vi "Teleop.vi"(10 "Match Info":T1={"Autonomous Elapsed Seconds"=0.0, "TeleOp Elapsed Seconds"=0.0, "Disabled Elapsed Seconds"=0.0, "Visited Autonomous"=FALSE, "Visited TeleOp"=FALSE, "Visited Disabled"=FALSE, "Autonomous Settings"={"Autonomous Style"=enum."Independent", "VI Refnum"=refnum}}, 11 "Call Context":T2) -> ()   [LabVIEW 2020]
doc: "This VI is called for each TeleOp packet received from the DS where the robot is not disabled. It is often used to read from the joysticks and update I/O or to update setpoints for timed control loops. It should complete and return within 20 milliseconds or it may miss DS packets."
uses:
  <vilib>/Rock Robotics/Network Tables/NT Write Numeric Array.vi
  <vilib>/Rock Robotics/Network Tables/NT Write Boolean Array.vi
  <vilib>/Rock Robotics/WPI/Joystick/XBox Buttons Indexer.ctl
  <vilib>/Rock Robotics/WPI/DriverStation/WPI_DriverStationMatch Info.ctl
  <vilib>/Rock Robotics/WPI/DriverStation/WPI_DriverStationDerivedRobotMode.ctl
panel:
  out "Right  Bumper?":bool
  out "Button  Y?":bool
  out "Button  X?":bool
  out "Button  B?":bool
  out "Left Bumper ?":bool
  out "Button A?":bool
  out "Motor Values":dbl[](array[numeric])
  out "Stick 2":dbl
  out "Stick 1":dbl
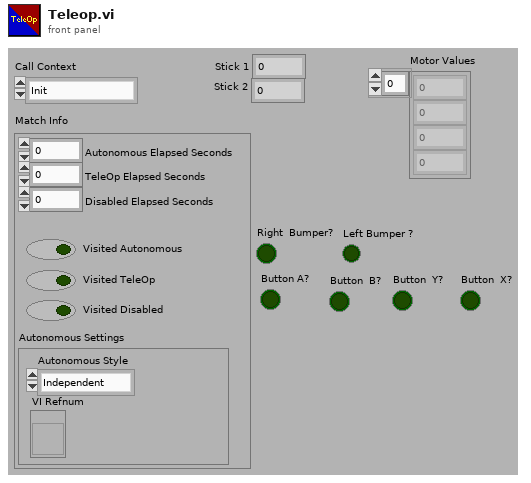
[diagram p1: front panel]
types:
  T1 = typedef "WPI_DriverStationMatch Info.ctl" = cluster{"Autonomous Elapsed Seconds":dbl, "TeleOp Elapsed Seconds":dbl, "Disabled Elapsed Seconds":dbl, "Visited Autonomous":bool, "Visited TeleOp":bool, "Visited Disabled":bool, "Autonomous Settings":cluster{"Autonomous Style":enum16{"Iterative", "Independent"}, "VI Refnum":refnum<vi>}}
  T2 = typedef "WPI_DriverStationDerivedRobotMode.ctl" = enum16{"Init", "Execute", "Stop"}
  T3 = typedef "XBox Buttons Indexer.ctl" = enum16{"A", "B", "X", "Y", "Left Bumper", "Right Bumper", "Back", "Start", "Left Joystick", "Right Joystick"}
  T4 = typedef "WPI_RobotDriveDevRef.ctl" = cluster{"DevStatus":errorcluster, "Motors[]":T5[], "Square Inputs":bool, "Max Output":dbl}
  T5 = typedef "WPI_MotorControlDeviceRef.ctl" = cluster{"DeviceStatus":errorcluster, "Type":T6, "PWM":cluster{"PWM Channel":T7, "DeadBand":T8}, "CAN":cluster{"Device Number":u8, "SetOutput VI Ref":variant, "GetOutput VI Ref":variant, "Enable VI Ref":variant, "Disable VI Ref":variant, "Data":variant}, "Invert":bool, "DIO PWM":cluster{"PWM \"Enable\" Channel":T7, "DIOChannel":T9, "PWM Rate":dbl}}
  T6 = typedef "WPI_MotorControlType.ctl" = enum16{"PWM", "CAN", "DIO PWM"}
  T7 = typedef "FPGA_DIOPWMChannel.ctl" = enum8{"PWM 0", "PWM 1", "PWM 2", "PWM 3", "PWM 4", "PWM 5", "PWM 6", "PWM 7", "PWM 8", "PWM 9", "PWM MXP 0", "PWM MXP 1", "PWM MXP 2", "PWM MXP 3", "PWM MXP 4", "PWM MXP 5", "PWM MXP 6", "PWM MXP 7", "PWM MXP 8", "PWM MXP 9", "Invalid"}
  T8 = typedef "WPI_PWMDeadband.ctl" = cluster{"Name":string, "maxPositivePwm":i32, "minPositivePwm":i32, "centerPwm":i32, "maxNegativePwm":i32, "minNegativePwm":i32, "angularRange":u16}
  T9 = typedef "FPGA_DIOChannel.ctl" = enum8{"DIO 0", "DIO 1", "DIO 2", "DIO 3", "DIO 4", "DIO 5", "DIO 6", "DIO 7", "DIO 8", "DIO 9", "DIO MXP 0", "DIO MXP 1", "DIO MXP 2", "DIO MXP 3", "DIO MXP 4", "DIO MXP 5", "DIO MXP 6", "DIO MXP 7", "DIO MXP 8", "DIO MXP 9", "DIO MXP 10", "DIO MXP 11", "DIO MXP 12", "DIO MXP 13", "DIO MXP 14", "DIO MXP 15", "SPI Port CS1", "SPI Port CS2", "SPI Port CS3", "SPI Port MISO", "SPI Port MOSI", "Invalid"}
  T10 = typedef "WPI_JoystickDevRef.ctl" = cluster{"Device":T11}
  T11 = typedef "WPI_JoystickDeviceEnum.ctl" = enum16{"USB 0", "USB 1", "USB 2", "USB 3", "USB 4", "USB 5"}
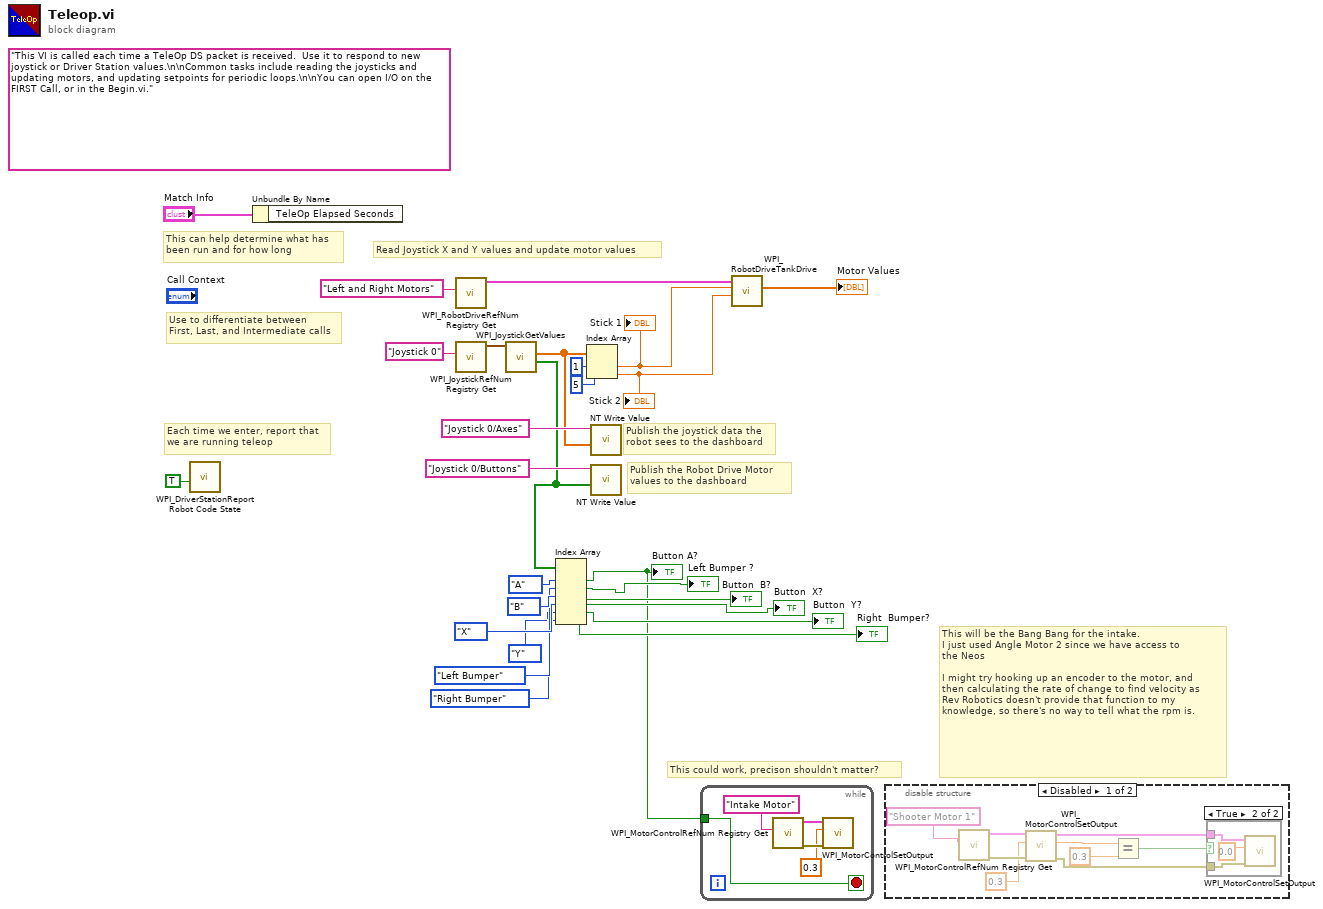
[diagram p0: block diagram]
diagram:
  (unwired) "This VI is called each time a TeleOp DS packet is received.  Use it to respond to new joystick or Driver Station values.\n\nCommon tasks include reading the joysticks and updating motors, and updating setpoints for periodic loops.\n\nYou can open I/O on the FIRST Call, or in the Begin.vi."
  # "This could work, precison shouldn't matter?"
  # "This will be the Bang Bang for the intake. \nI just used Angle Motor 2 since we have access to \nthe Neos\n\nI might try hooking up an encoder to the motor, and \nthen calculating the rate of change to find velocity as \nRev Robotics doesn't provide that function to my \nknowledge, so there's no way to tell what the rpm is."
  # "Publish the Robot Drive Motor\nvalues to the dashboard"
  # "Publish the joystick data the\nrobot sees to the dashboard"
  # "Each time we enter, report that\nwe are running teleop"
  # "Use to differentiate between\nFirst, Last, and Intermediate calls"
  # "This can help determine what has\nbeen run and for how long"
  # "Read Joystick X and Y values and update motor values"
  n1 = call <vilib>:"WPI_DriverStationReport Robot Code State.vi"("TeleOp"=TRUE ("Autonomous")) -> ()  [unwired: 10 in, 1 out]
  n2 = Unbundle By Name("Match Info") -> ()  [unwired: 1 out]
  n3 = call <vilib>:"WPI_RobotDriveRefNum Registry Get.vi"("refnum name"="Left and Right Motors") -> ("RobotDriveDevRef"=w17:T4)  [unwired: 1 in, 9 out]
  n4 = call <vilib>:"WPI_JoystickRefNum Registry Get.vi"("refnum name"="Joystick 0") -> ("JoystickDevRef"=w24:T10)  [unwired: 1 in, 9 out]
  n5 = call <vilib>:"WPI_JoystickGetValues.vi"("JoystickDevRef"=w24) -> ("Buttons"=w13:bool[], "Axes"=w20:dbl[])  [unwired: 6 in, 3 out]
  n6 = Index Array(array=w13, index #1=XBox_Buttons_Indexer."A" ("XBox Buttons"), index #2=XBox_Buttons_Indexer."Left Bumper" ("XBox Buttons"), index #3=XBox_Buttons_Indexer."B" ("XBox Buttons"), index #4=XBox_Buttons_Indexer."X" ("XBox Buttons"), index #5=XBox_Buttons_Indexer."Y" ("XBox Buttons"), index #6=XBox_Buttons_Indexer."Right Bumper" ("XBox Buttons")) -> (element #1=w1:bool, element #2=→"Left Bumper ?":bool, element #3=→"Button  B?":bool, element #4=→"Button  X?":bool, element #5=→"Button  Y?":bool, element #6=→"Right  Bumper?":bool)
  "Button A?" <- w1
  n7 = Index Array(array=w20, index #1=1 ("index"), index #2=5 ("index")) -> (element #1=w16:dbl, element #2=w15:dbl)
  "Stick 1" <- w16
  "Stick 2" <- w15
  n8 = call-poly <vilib>:"NT Write Value.vi"("Numeric Array"=w20, "Name"="Joystick 0/Axes") -> ()  [unwired: 9 in, 1 out]
  n9 = call-poly <vilib>:"NT Write Value.vi"("Boolean Array"=w13, "Name"="Joystick 0/Buttons") -> ()  [unwired: 9 in, 1 out]
  n10 = while {
    tunnel: w1 -> [w28]
    stop <- w28 stop-if-true
    n11 = call <vilib>:"WPI_MotorControlRefNum Registry Get.vi"("refnum name"="Intake Motor") -> ("error out"=w30:errorcluster, "MotorControlDevRef"=w31:T5)  [unwired: 9 in]
    n12 = call <vilib>:"WPI_MotorControlSetOutput.vi"("error in (no error)"=w30, "Output"=0.3, "MotorControlDevRef"=w31) -> ()  [unwired: 6 in, 3 out]
  }
  n13 = call <vilib>:"WPI_RobotDriveTankDrive.vi"("Right axis value"=w15, "Left axis value"=w16, "RobotDriveDevRef"=w17) -> ("Motor Values"=→"Motor Values":dbl[])  [unwired: 6 in, 2 out]
  n14 = disable-structure shown="Disabled" {
    frame Disabled {
      n15 = call <vilib>:"WPI_MotorControlRefNum Registry Get.vi"("refnum name"="Shooter Motor 1") -> ("error out"=w37:errorcluster, "MotorControlDevRef"=w36:T5)  [unwired: 9 in]
      n16 = call <vilib>:"WPI_MotorControlSetOutput.vi"("error in (no error)"=w37, "Output"=0.3, "MotorControlDevRef"=w36) -> ("error out"=w39:errorcluster, "Motor Output"=w40:dbl, "MotorControlDevRef"=w41:T5)  [unwired: 6 in]
      n17 = Equal?(x=w40, y=0.3 ("Output")) -> (x = y?=w38:bool)
      n18 = case shown="True" w38 {
        tunnel: w41 -> [_ w44]
        tunnel: w39 -> [_ w43]
        frame False {
        }
        frame True {
          n19 = call <vilib>:"WPI_MotorControlSetOutput.vi"("error in (no error)"=w43, "Output"=0.0, "MotorControlDevRef"=w44) -> ()  [unwired: 6 in, 3 out]
        }
      }
    }
    frame Enabled {
    }
  }
